vi "ErrorControlMissing.vi"(0 "Create Error?":bool, 5 "Control Name":string, 11 "error in":errorcluster) -> (15 "error out":errorcluster)   [LabVIEW 2016]
doc: "Creates error if the control is not found."
uses:
  <vilib>/Utility/error.llb/Error Cluster From Error Code.vi
  <vilib>/ErrorRing/Error Ring.xnode
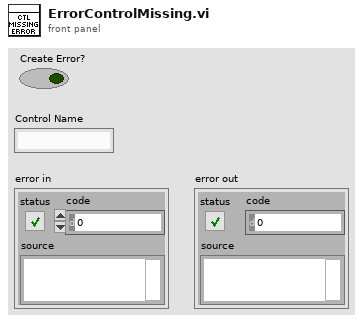
[diagram p1: front panel]
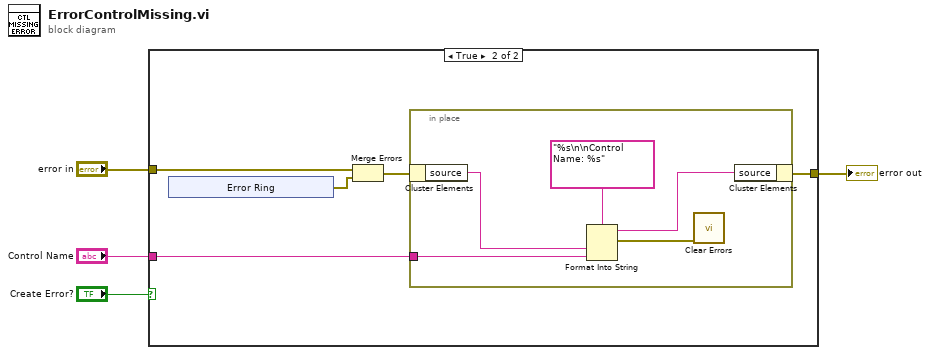
[diagram p0: block diagram]
diagram:
  n1 = case shown="True" "Create Error?" {
    tunnel: "error in" -> [w5 w10]
    tunnel: [w5 w7] -> w3
    tunnel: "Control Name" -> [_ w6]
    frame False {
    }
    frame True {
      n2 = xnode "Error Ring"() -> ("error out"=w9:errorcluster)
      n3 = Merge Errors(w10, w9) -> (w8:errorcluster)
      n4 = in-place {
        in-place-border: w6 -> [w15]
        n5 = in-place-cluster #1(w8) -> ("source"=w12:string)
        n6 = Format Into String(format string="%s\n\nControl Name: %s", w12, w15) -> (resulting string=w13:string, error out=w11:errorcluster)  [unwired: 2 in]
        n7 = call <vilib>:"Clear Errors.vi"("error in (no error)"=w11) -> ()  [unwired: 5 in, 2 out]
        n8 = in-place-cluster #1("source"=w13) -> (w7:errorcluster)
      }
    }
  }
  "error out" <- w3
